vi "GetDateTimeArray.vi"() -> (0 "DateTime array":string[](array[string]))   [LabVIEW 2023]
panel:
  out "resulting Data string":string
  out "resulting Time string":string
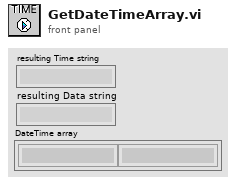
[diagram p1: front panel]
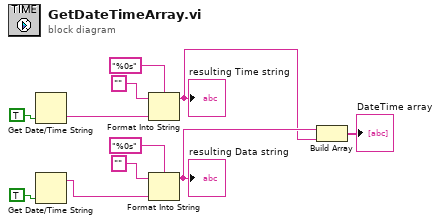
[diagram p0: block diagram]
diagram:
  n1 = Get Date/Time String(want seconds? (F)=TRUE) -> (time string=w9:string)  [unwired: 2 in, 1 out]
  n2 = Get Date/Time String(want seconds? (F)=TRUE) -> (date string=w4:string)  [unwired: 2 in, 1 out]
  n3 = Format Into String(format string="%0s", initial string="", w9) -> (resulting string=w2:string)  [unwired: 1 in, 1 out]
  "resulting Time string" <- w2
  n4 = Format Into String(format string="%0s", initial string="", w4) -> (resulting string=w3:string)  [unwired: 1 in, 1 out]
  "resulting Data string" <- w3
  n5 = Build Array(w3, w2) -> (→"DateTime array":string[])
